vi "Setup CurrentSource.vi"(6 "Source":T1(ring), 8 "error in (no error)":errorcluster, 11 "VISA Refnum in":refnum<visa-resource-name>="B2901_SourceMeter") -> (0 "error out":errorcluster, 2 "task out":refnum<k24>, 3 "VISA Refnum out":refnum<visa-resource-name>)   [LabVIEW 2024]
uses:
  <instrlib>/ULx/ULx_LV.dll
  Documents/LabVIEW Data/TestHarnessDPL_v24/Program Files/National Instruments/LabVIEW 2024/instr.lib/Keithley 24XX/Keithley 24XX.lvlib
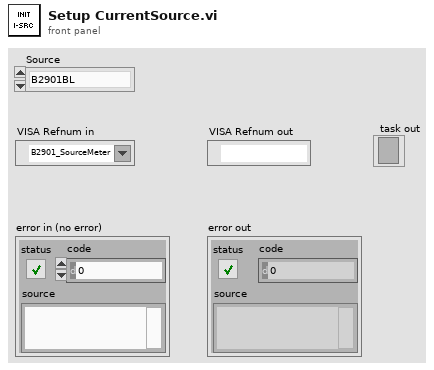
[diagram p1: front panel]
types:
  T1 = enum16{"B2901BL", "USB-3104 10M o/p3", "USB-3104 100K o/p5"}
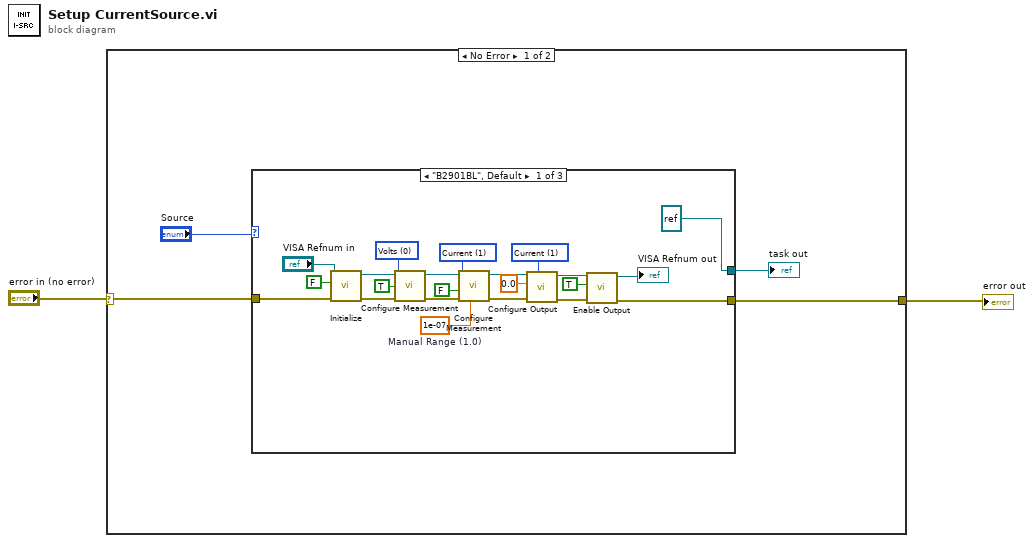
[diagram p0: block diagram]
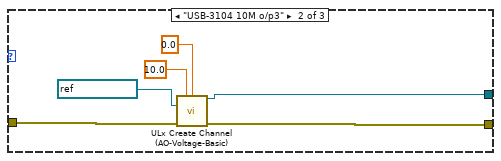
[diagram p2: hidden frame]
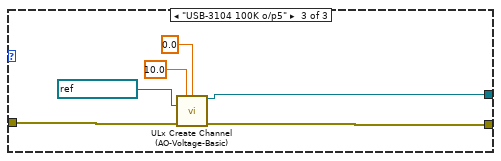
[diagram p3: hidden frame]
diagram:
  n1 = case shown="No Error" "error in (no error)" {
    selector: "error in (no error)" -> [w5 w41]
    tunnel: [w6 w41] -> w2
    frame No Error {
      n2 = case shown="\"B2901BL\", Default" "Source" {
        tunnel: [w23 w32 w38] -> w6
        tunnel: w5 -> [w8 w33 w39]
        tunnel: [refnum<k24> refnum ("task out") w29 w35] -> w3
        frame "B2901BL", Default {
          w28 = u16 0 items=["Volts", "Current", "Resistance"] ("Function (0: Volts)")
          w17 = u16 1 items=["Voltage", "Current"] ("Source Mode  (0: Voltage)")
          w26 = 1e-07  # Manual Range (1.0)
          w13 = u16 1 items=["Volts", "Current", "Resistance"] ("Function (0: Volts)")
          n3 = call "Initialize.vi"("error in (no error)"=w8, "ID Query (True)"=FALSE, "VISA resource name"="VISA Refnum in") -> ("error out"=w25:errorcluster, "VISA resource name out"=w24:refnum<visa-resource-name>)  [unwired: 7 in]
          n4 = call "Configure Measurement.vi"("error in (no error)"=w25, "Enable Auto Range (T:Enable)"=TRUE ("Enable Voltage Measurement (T: Enable)"), "Function (0: Volts)"=w28, "VISA resource name"=w24) -> ("error out"=w12:errorcluster, "VISA resource name out"=w11:refnum<visa-resource-name>)  [unwired: 6 in]
          n5 = call "Configure Measurement.vi"("Manual Range (1.0)"=w26, "error in (no error)"=w12, "Enable Auto Range (T:Enable)"=FALSE, "Function (0: Volts)"=w13, "VISA resource name"=w11) -> ("error out"=w15:errorcluster, "VISA resource name out"=w16:refnum<visa-resource-name>)  [unwired: 5 in]
          n6 = call "Configure Output.vi"("Source Mode  (0: Voltage)"=w17, "error in (no error)"=w15, "Output Level (0)"=0.0, "VISA resource name"=w16) -> ("error out"=w19:errorcluster, "VISA resource name out"=w20:refnum<visa-resource-name>)  [unwired: 6 in]
          n7 = call "Enable Output.vi"("error in (no error)"=w19, "Enable Output (T: Enable)"=TRUE, "VISA resource name"=w20) -> ("error out"=w23:errorcluster, "VISA resource name out"=→"VISA Refnum out":refnum<visa-resource-name>)  [unwired: 7 in]
        }
        frame "USB-3104 10M o/p3" {
          n8 = call <instrlib>:"ULx Create Channel (AO-Voltage-Basic).vi"("maximum value"=10.0, "minimum value"=0.0, "physical channels"=refnum<k21> "Dev0/Ao3", "error in"=w33) -> ("task out"=w29:refnum<k24>, "error out"=w32:errorcluster)  [unwired: 10 in]
        }
        frame "USB-3104 100K o/p5" {
          n9 = call <instrlib>:"ULx Create Channel (AO-Voltage-Basic).vi"("maximum value"=10.0, "minimum value"=0.0, "physical channels"=refnum<k21> "Dev0/Ao5", "error in"=w39) -> ("task out"=w35:refnum<k24>, "error out"=w38:errorcluster)  [unwired: 10 in]
        }
      }
      "task out" <- w3
    }
    frame Error {
    }
  }
  "error out" <- w2
